vi "tap_stimulus_setup.vi"(1 "input cluster":T1) -> (0 "output cluster":T2)   [LabVIEW 2015]
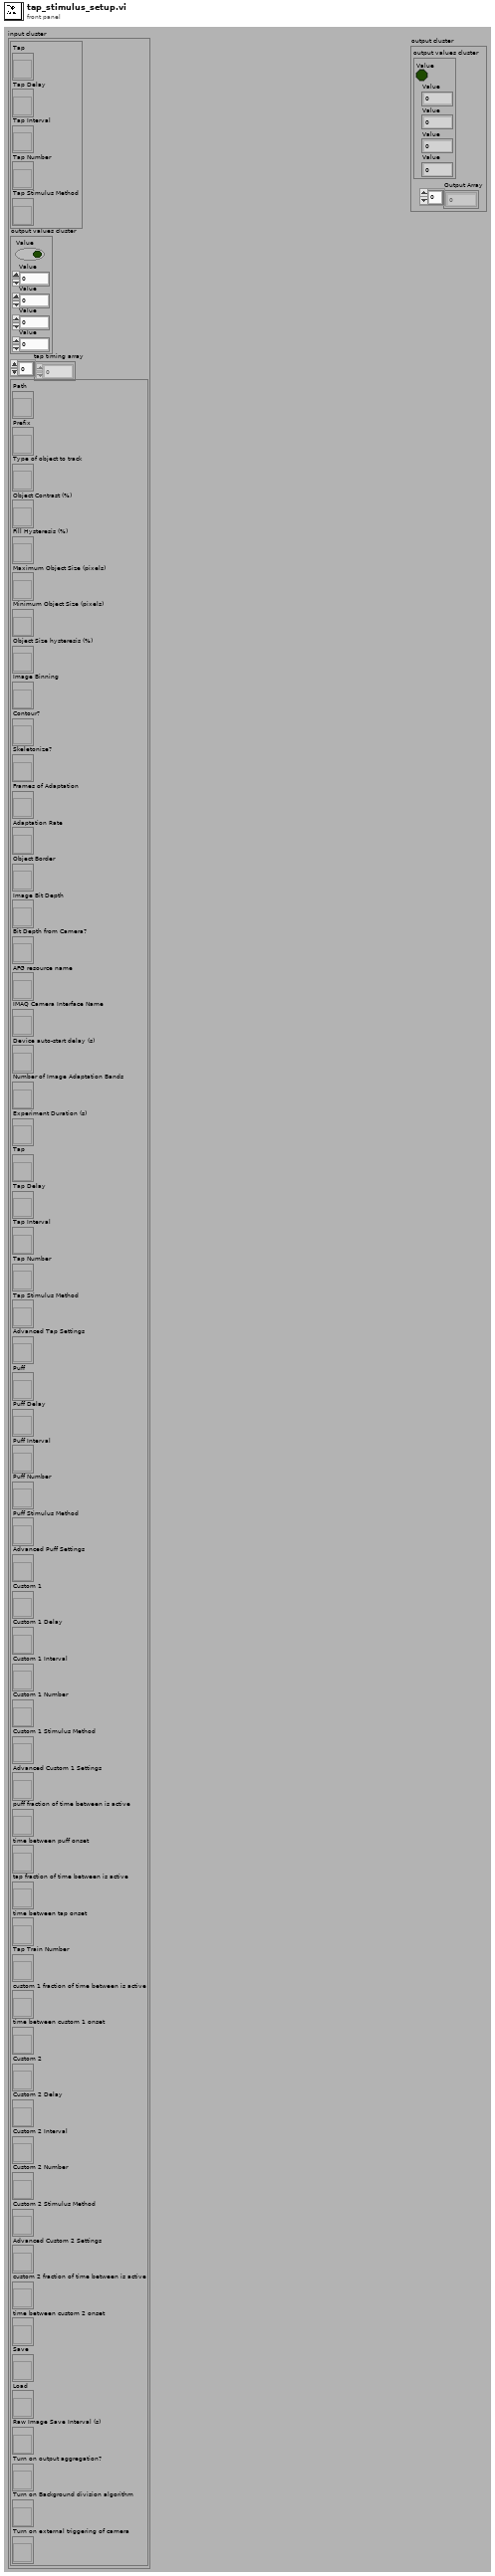
[diagram p1: front panel]
types:
  T1 = cluster{cluster{"Tap":refnum<vi>, "Tap Delay":refnum<vi>, "Tap Interval":refnum<vi>, "Tap Number":refnum<vi>, "Tap Stimulus Method":refnum<vi>}, "output values cluster":cluster{"Value":bool, "Value":dbl, "Value":dbl, "Value":dbl, "Value":u16}, "tap timing array":dbl[], cluster{"Path":refnum<vi>, "Prefix":refnum<vi>, "Type of object to track":refnum<vi>, "Object Contrast (%)":refnum<vi>, "Fill Hysteresis (%)":refnum<vi>, "Maximum Object Size (pixels)":refnum<vi>, "Minimum Object Size (pixels)":refnum<vi>, "Object Size hysteresis (%)":refnum<vi>, "Image Binning":refnum<vi>, "Contour?":refnum<vi>, "Skeletonize?":refnum<vi>, "Frames of Adaptation":refnum<vi>, "Adaptation Rate":refnum<vi>, "Object Border":refnum<vi>, "Image Bit Depth":refnum<vi>, "Bit Depth from Camera?":refnum<vi>, "AFG resource name":refnum<vi>, "IMAQ Camera Interface Name":refnum<vi>, "Device auto-start delay (s)":refnum<vi>, "Number of Image Adaptation Bands":refnum<vi>, "Experiment Duration (s)":refnum<vi>, "Tap":refnum<vi>, "Tap Delay":refnum<vi>, "Tap Interval":refnum<vi>, "Tap Number":refnum<vi>, "Tap Stimulus Method":refnum<vi>, "Advanced Tap Settings":refnum<vi>, "Puff":refnum<vi>, "Puff Delay":refnum<vi>, "Puff Interval":refnum<vi>, "Puff Number":refnum<vi>, "Puff Stimulus Method":refnum<vi>, "Advanced Puff Settings":refnum<vi>, "Custom 1":refnum<vi>, "Custom 1 Delay":refnum<vi>, "Custom 1 Interval":refnum<vi>, "Custom 1 Number":refnum<vi>, "Custom 1 Stimulus Method":refnum<vi>, "Advanced Custom 1 Settings":refnum<vi>, "puff fraction of time between is active":refnum<vi>, "time between puff onset":refnum<vi>, "tap fraction of time between is active":refnum<vi>, "time between tap onset":refnum<vi>, "Tap Train Number":refnum<vi>, "custom 1 fraction of time between is active":refnum<vi>, "time between custom 1 onset":refnum<vi>, "Custom 2":refnum<vi>, "Custom 2 Delay":refnum<vi>, "Custom 2 Interval":refnum<vi>, "Custom 2 Number":refnum<vi>, "Custom 2 Stimulus Method":refnum<vi>, "Advanced Custom 2 Settings":refnum<vi>, "custom 2 fraction of time between is active":refnum<vi>, "time between custom 2 onset":refnum<vi>, "Save":refnum<vi>, "Load":refnum<vi>, "Raw Image Save Interval (s)":refnum<vi>, "Turn on output aggregation?":refnum<vi>, "Turn on Background division algorithm":refnum<vi>, "Turn on external triggering of camera":refnum<vi>}}
  T2 = cluster{"output values cluster":cluster{"Value":bool, "Value":dbl, "Value":dbl, "Value":dbl, "Value":u16}, "Output Array":dbl[]}
  T3 = cluster{"Tap":refnum<vi>, "Tap Delay":refnum<vi>, "Tap Interval":refnum<vi>, "Tap Number":refnum<vi>, "Tap Stimulus Method":refnum<vi>}
  T4 = cluster{"Value":bool, "Value":dbl, "Value":dbl, "Value":dbl, "Value":u16}
  T5 = cluster{"Path":refnum<vi>, "Prefix":refnum<vi>, "Type of object to track":refnum<vi>, "Object Contrast (%)":refnum<vi>, "Fill Hysteresis (%)":refnum<vi>, "Maximum Object Size (pixels)":refnum<vi>, "Minimum Object Size (pixels)":refnum<vi>, "Object Size hysteresis (%)":refnum<vi>, "Image Binning":refnum<vi>, "Contour?":refnum<vi>, "Skeletonize?":refnum<vi>, "Frames of Adaptation":refnum<vi>, "Adaptation Rate":refnum<vi>, "Object Border":refnum<vi>, "Image Bit Depth":refnum<vi>, "Bit Depth from Camera?":refnum<vi>, "AFG resource name":refnum<vi>, "IMAQ Camera Interface Name":refnum<vi>, "Device auto-start delay (s)":refnum<vi>, "Number of Image Adaptation Bands":refnum<vi>, "Experiment Duration (s)":refnum<vi>, "Tap":refnum<vi>, "Tap Delay":refnum<vi>, "Tap Interval":refnum<vi>, "Tap Number":refnum<vi>, "Tap Stimulus Method":refnum<vi>, "Advanced Tap Settings":refnum<vi>, "Puff":refnum<vi>, "Puff Delay":refnum<vi>, "Puff Interval":refnum<vi>, "Puff Number":refnum<vi>, "Puff Stimulus Method":refnum<vi>, "Advanced Puff Settings":refnum<vi>, "Custom 1":refnum<vi>, "Custom 1 Delay":refnum<vi>, "Custom 1 Interval":refnum<vi>, "Custom 1 Number":refnum<vi>, "Custom 1 Stimulus Method":refnum<vi>, "Advanced Custom 1 Settings":refnum<vi>, "puff fraction of time between is active":refnum<vi>, "time between puff onset":refnum<vi>, "tap fraction of time between is active":refnum<vi>, "time between tap onset":refnum<vi>, "Tap Train Number":refnum<vi>, "custom 1 fraction of time between is active":refnum<vi>, "time between custom 1 onset":refnum<vi>, "Custom 2":refnum<vi>, "Custom 2 Delay":refnum<vi>, "Custom 2 Interval":refnum<vi>, "Custom 2 Number":refnum<vi>, "Custom 2 Stimulus Method":refnum<vi>, "Advanced Custom 2 Settings":refnum<vi>, "custom 2 fraction of time between is active":refnum<vi>, "time between custom 2 onset":refnum<vi>, "Save":refnum<vi>, "Load":refnum<vi>, "Raw Image Save Interval (s)":refnum<vi>, "Turn on output aggregation?":refnum<vi>, "Turn on Background division algorithm":refnum<vi>, "Turn on external triggering of camera":refnum<vi>}
  T6 = cluster{"tap fraction of time between is active":refnum<vi>, "time between tap onset":refnum<vi>, "Tap Train Number":refnum<vi>}
  T7 = cluster{"Value":bool, "Value":dbl, "Value":dbl, "Value":i32, "Value":u16}
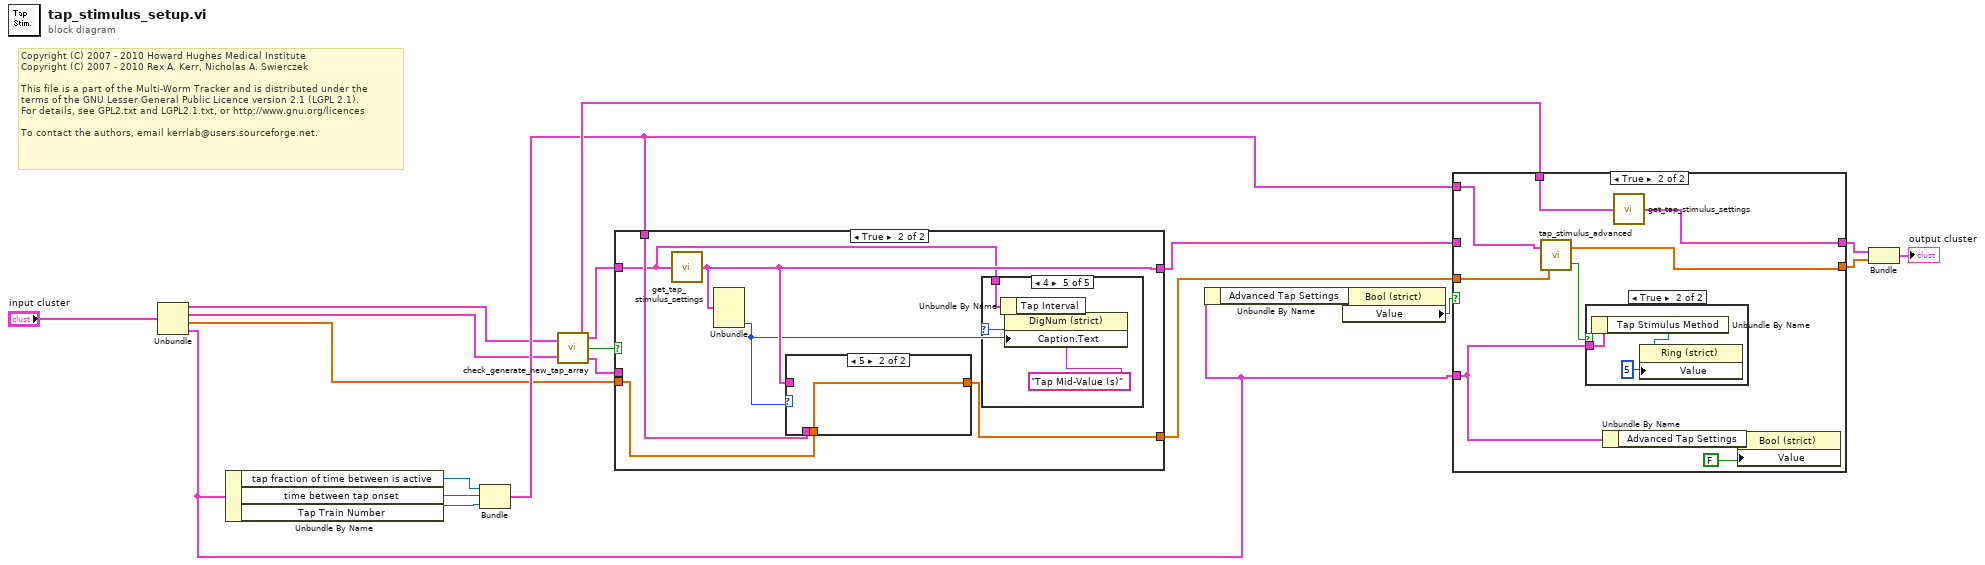
[diagram p0: block diagram]
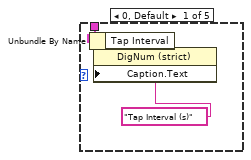
[diagram p3: hidden frame]
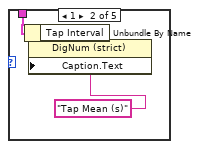
[diagram p4: hidden frame]
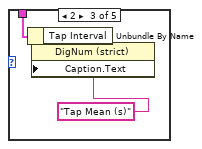
[diagram p5: hidden frame]
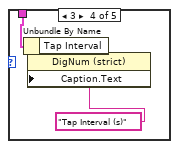
[diagram p6: hidden frame]
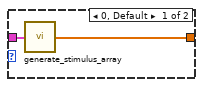
[diagram p7: hidden frame]
diagram:
  # "Copyright (C) 2007 - 2010 Howard Hughes Medical Institute\nCopyright (C) 2007 - 2010 Rex A. Kerr, Nicholas A. Swierczek\n \nThis file is a part of the Multi-Worm Tracker and is distributed under the\nterms of the GNU Lesser General Public Licence version 2.1 (LGPL 2.1).\nFor details, see GPL2.txt and LGPL2.1.txt, or http://www.gnu.org/licences\n \nTo contact the authors, email kerrlab@users.sourceforge.net."
  n1 = Unbundle("input cluster") -> (w8:T3, "output values cluster"=w9:T4, "tap timing array"=w10:dbl[], w2:T5)
  n2 = Unbundle By Name(w2) -> ("tap fraction of time between is active"=w14:refnum<vi>, "time between tap onset"=w13:refnum<vi>, "Tap Train Number"=w12:refnum<vi>)
  n3 = Bundle("tap fraction of time between is active"=w14, "time between tap onset"=w13, "Tap Train Number"=w12) -> (w11:T6)  [unwired: 1 in]
  n4 = call "check_generate_new_tap_array.vi"("Input References Cluster"=w8, "Input values cluster"=w9) -> ("Output References Cluster"=w15:T3, "Need new tap array?"=w18:bool, "Output Values Cluster"=w17:T7)
  n5 = case shown="True" w18 {
    tunnel: [w21 w27] -> w19
    tunnel: w10 -> [w21 w24]
    tunnel: w15 -> [_ w22]
    tunnel: [w20 w26] -> w16
    tunnel: w17 -> [w20 _]
    tunnel: w11 -> [_ w25]
    frame False {
    }
    frame True {
      n6 = call "get_tap_stimulus_settings.vi"("Input References Cluster"=w22) -> ("output values cluster"=w26:T4)
      n7 = Unbundle(w26) -> ("Value"=w23:u16)  [unwired: 4 out]
      n8 = case shown="5" w23 {
        tunnel: [w44 w45] -> w27
        tunnel: w26 -> [w43 _]
        tunnel: w25 -> [_ _]
        tunnel: w24 -> [_ w45]
        frame 0, Default {
          n9 = call "generate_stimulus_array.vi"("Values Cluster"=w43) -> ("Array"=w44:dbl[])
        }
        frame 5 {
        }
      }
      n10 = case shown="4" w23 {
        tunnel: w22 -> [w30 w32 w34 w37 w40]
        frame 0, Default {
          n11 = Unbundle By Name(w30) -> ("Tap Interval"=w29:refnum<vi>)
          n12 = property class="DigNum (strict)"(reference=w29, "Caption.Text"="Tap Interval (s)") -> ()  [unwired: 1 in, 2 out]
        }
        frame 1 {
          n13 = Unbundle By Name(w32) -> ("Tap Interval"=w33:refnum<vi>)
          n14 = property class="DigNum (strict)"(reference=w33, "Caption.Text"="Tap Mean (s)") -> ()  [unwired: 1 in, 2 out]
        }
        frame 2 {
          n15 = Unbundle By Name(w34) -> ("Tap Interval"=w36:refnum<vi>)
          n16 = property class="DigNum (strict)"(reference=w36, "Caption.Text"="Tap Mean (s)") -> ()  [unwired: 1 in, 2 out]
        }
        frame 3 {
          n17 = Unbundle By Name(w37) -> ("Tap Interval"=w39:refnum<vi>)
          n18 = property class="DigNum (strict)"(reference=w39, "Caption.Text"="Tap Interval (s)") -> ()  [unwired: 1 in, 2 out]
        }
        frame 4 {
          n19 = Unbundle By Name(w40) -> ("Tap Interval"=w42:refnum<vi>)
          n20 = property class="DigNum (strict)"(reference=w42, "Caption.Text"="Tap Mid-Value (s)") -> ()  [unwired: 1 in, 2 out]
        }
      }
    }
  }
  n21 = Unbundle By Name(w2) -> ("Advanced Tap Settings"=w4:refnum<vi>)
  n22 = property class="Bool (strict)"(reference=w4) -> ("Value"=w3:bool)  [unwired: 1 in, 2 out]
  n23 = case shown="True" w3 {
    tunnel: [w47 w54] -> w6
    tunnel: w19 -> [w47 w56]
    tunnel: w2 -> [_ w49]
    tunnel: w11 -> [_ w55]
    tunnel: w16 -> [w46 _]
    tunnel: [w46 w53] -> w7
    tunnel: w15 -> [_ w52]
    frame False {
    }
    frame True {
      n24 = call "tap_stimulus_advanced.vi"("Input Array"=w56, "Cluster"=w55) -> ("Timing array changed?"=w48:bool, "Output Array"=w54:dbl[])
      n25 = case shown="True" w48 {
        tunnel: w49 -> [_ w59]
        frame False {
        }
        frame True {
          n26 = Unbundle By Name(w59) -> ("Tap Stimulus Method"=w58:refnum<vi>)
          n27 = property class="Ring (strict)"(reference=w58, "Value"=u16 5) -> ()  [unwired: 1 in, 2 out]
        }
      }
      n28 = Unbundle By Name(w49) -> ("Advanced Tap Settings"=w51:refnum<vi>)
      n29 = call "get_tap_stimulus_settings.vi"("Input References Cluster"=w52) -> ("output values cluster"=w53:T4)
      n30 = property class="Bool (strict)"(reference=w51, "Value"=FALSE) -> ()  [unwired: 1 in, 2 out]
    }
  }
  n31 = Bundle("output values cluster"=w7, "Output Array"=w6) -> (→"output cluster":T2)  [unwired: 1 in]
